vi "Read model_name.vi"(8 "error in (no error)":errorcluster, 11 "llm_anthropic_chatmodels in":refnum<class "llm_anthropic_chatmodels.lvclass">) -> (0 "error out":errorcluster, 2 "model_name":string(combo)="claude-3-5-sonnet-20240620", 3 "llm_anthropic_chatmodels out":refnum<class "llm_anthropic_chatmodels.lvclass">)   [LabVIEW 2020, in "llm_anthropic_chatmodels.lvclass"]
uses:
  llm_anthropic_chatmodels.lvclass
  llm_anthropic_chatmodels.lvclass/llm_anthropic_chatmodels.ctl
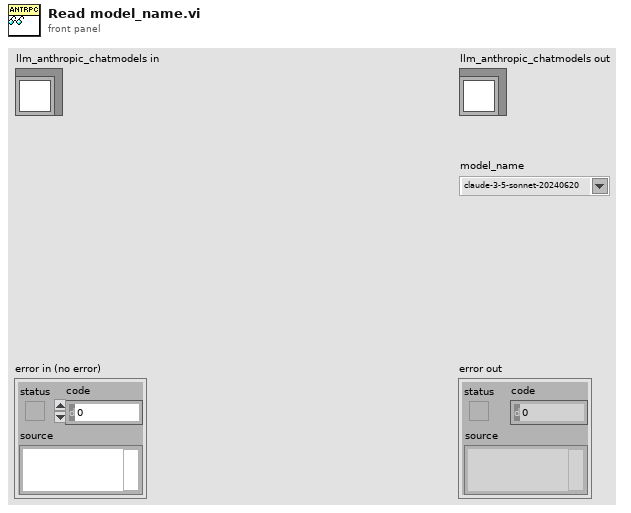
[diagram p1: front panel]
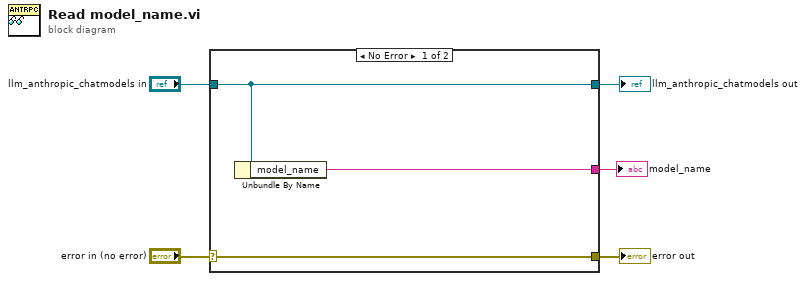
[diagram p0: block diagram]
diagram:
  n1 = case shown="No Error" "error in (no error)" {
    selector: "error in (no error)" -> [w8 w9]
    tunnel: [w8 w9] -> w4
    tunnel: [w7 w10] -> w2
    tunnel: "llm_anthropic_chatmodels in" -> [w7 w10]
    tunnel: [w6 _] -> w1
    frame No Error {
      n2 = Unbundle By Name(w7) -> ("model_name"=w6:string)
    }
    frame Error {
    }
  }
  "error out" <- w4
  "llm_anthropic_chatmodels out" <- w2
  "model_name" <- w1
